vi "Measurement UI.vi"() -> ()   [LabVIEW 2021, in "Table and Multicolumn Listbox.lvlib"]
uses:
  Table and Multicolumn Listbox.lvlib
panel:
  in  "Tab Control":enum32{"Table", "Multicolumn Listbox"}(tab)
  out "Table":string[][](table)
  out "Multicolumn Listbox":i32(listbox)
  in  "Value to be Inserted":string
  in  "Update":bool
  in  "Cell Coordinates":cluster{"Row":i32, "Column":i32}
  in  "Clear":bool
  # "Source: https://forums.ni.com/t5/Example-Code/Programmatically-Write-Values-to-a-Multicolumn-Listbox/ta-p/3495593"
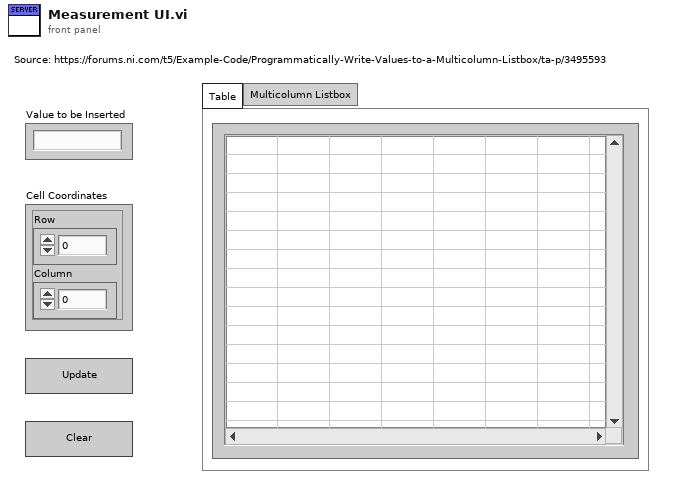
[diagram p1: front panel]
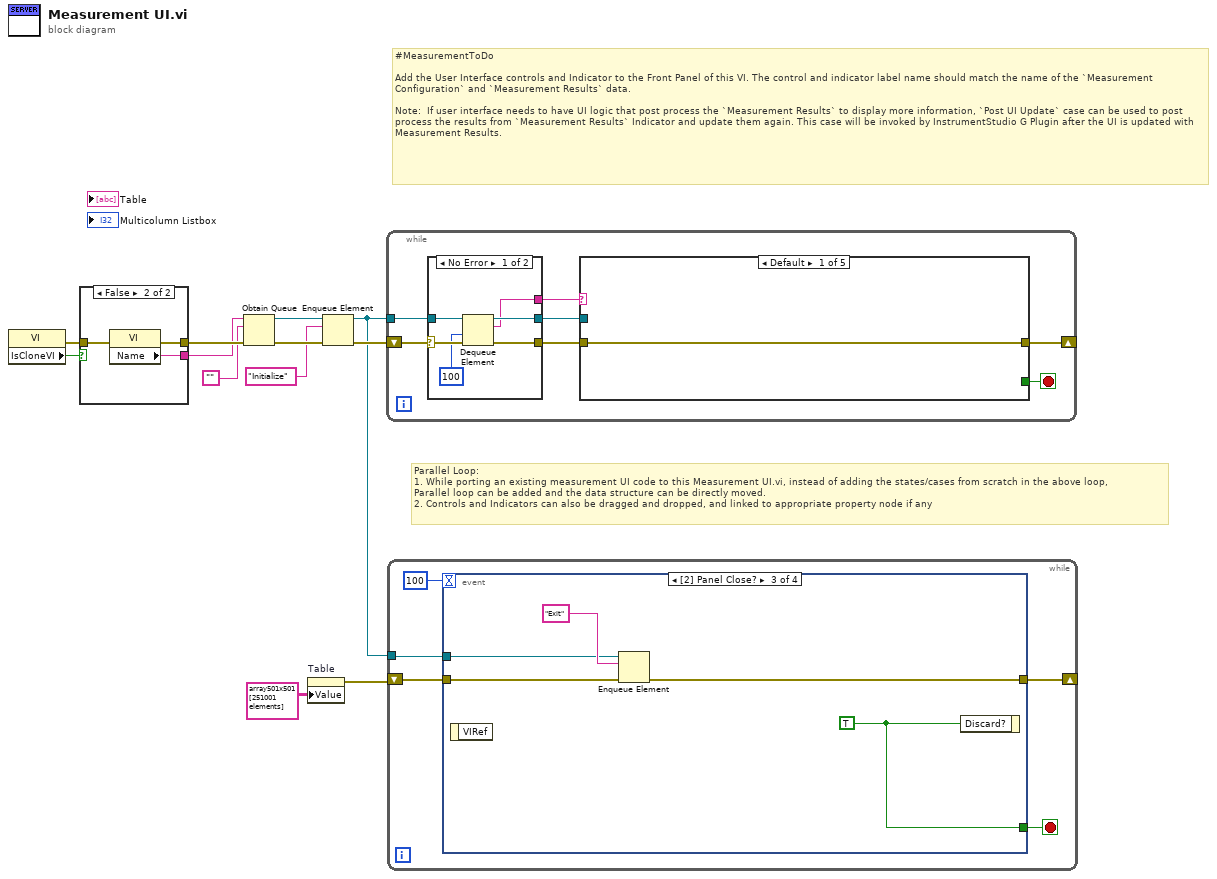
[diagram p0: block diagram]
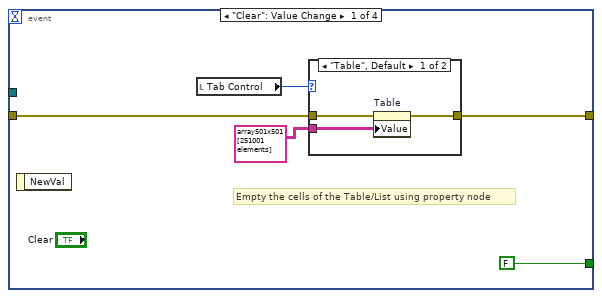
[diagram p2: hidden frame]
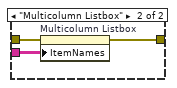
[diagram p3: hidden frame]
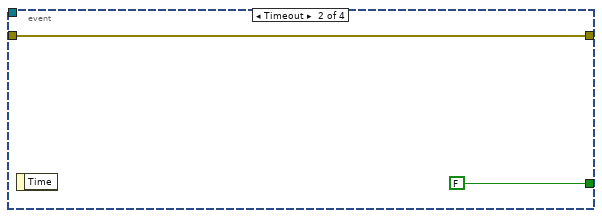
[diagram p4: hidden frame]
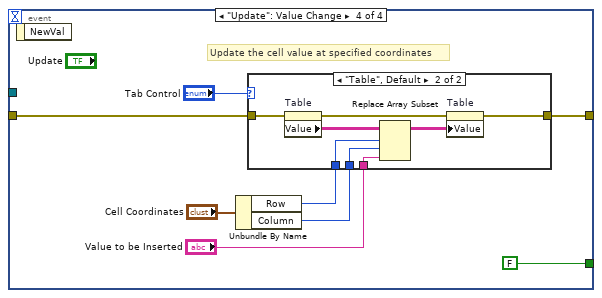
[diagram p5: hidden frame]
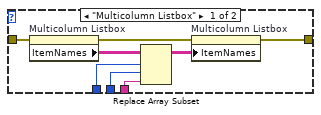
[diagram p6: hidden frame]
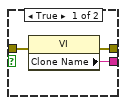
[diagram p7: hidden frame]
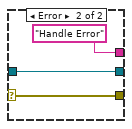
[diagram p8: hidden frame]
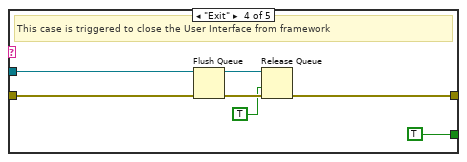
[diagram p11: hidden frame]
diagram:
  # "Parallel Loop:\n1. While porting an existing measurement UI code to this Measurement UI.vi, instead of adding the states/cases from scratch in the above loop,\nParallel loop can be added and the data structure can be directly moved.\n2. Controls and Indicators can also be dragged and dropped, and linked to appropriate property node if any"
  # "#MeasurementToDo  \n\nAdd the User Interface controls and Indicator to the Front Panel of this VI. The control and indicator label name should match the name of the `Measurement Configuration` and `Measurement Results` data.\n\nNote:  If user interface needs to have UI logic that post process the `Measurement Results` to display more information, `Post UI Update` case can be used to post process the results from `Measurement Results` Indicator and update them again. This case will be invoked by InstrumentStudio G Plugin after the UI is updated with Measurement Results."
  n1 = property class="VI"() -> (error out=w4:errorcluster, "IsCloneVI"=w5:bool)  [unwired: 2 in, 1 out]
  n2 = case shown="False" w5 {
    tunnel: [w15 w18] -> w12
    tunnel: [w14 w17] -> w11
    tunnel: w4 -> [w13 w16]
    frame True {
      n3 = property class="VI"(error in=w13) -> (error out=w15:errorcluster, "Clone Name"=w14:string)  [unwired: 1 in, 1 out]
    }
    frame False {
      n4 = property class="VI"(error in=w16) -> (error out=w18:errorcluster, "Name"=w17:string)  [unwired: 1 in, 1 out]
    }
  }
  n5 = Obtain Queue(name (unnamed)=w11, element data type="", error in (no error)=w12) -> (queue out=w8:refnum<queue>, error out=w10:errorcluster)  [unwired: 2 in, 1 out]
  n6 = property on="Table" class="Tbl (strict)"("Value"=string[][] array501x501[251001 elements] ("Table")) -> (error out=w2:errorcluster)  [unwired: 2 in, 1 out]
  n7 = Enqueue Element(queue=w8, element="Initialize", error in (no error)=w10) -> (queue out=w3:refnum<queue>, error out=w9:errorcluster)  [unwired: 1 in, 1 out]
  n8 = while {
    shift-right: [w20] -> _
    shift-left: w9 -> [w25]
    tunnel: w3 -> [w23]
    stop <- w19 stop-if-true
    n9 = case shown="No Error" w25 {
      selector: w25 -> [w31 w34]
      tunnel: [w30 w34] -> w24
      tunnel: w23 -> [w29 w33]
      tunnel: [w28 w33] -> w22
      tunnel: [w27 "Handle Error"] -> w21
      frame No Error {
        n10 = Dequeue Element(queue=w29, timeout in ms (-1)=100, error in (no error)=w31) -> (queue out=w28:refnum<queue>, element=w27:string, error out=w30:errorcluster)  [unwired: 1 out]
      }
      frame Error {
      }
    }
    n11 = case shown="Default" w21 {
      tunnel: w24 -> [w35 w36 w37 w44 w45]
      tunnel: w22 -> [_ _ _ w42 _]
      tunnel: [w35 w36 w37 w39 w45] -> w20
      tunnel: [_ _ _ TRUE _] -> w19
      frame Default {
      }
      frame "Initialize" {
      }
      frame "Post UI Update" {
        # "This case will be triggered, after framework updates the User interface with result values."
      }
      frame "Exit" {
        # "This case is triggered to close the User Interface from framework"
        n12 = Flush Queue(queue=w42, error in (no error)=w44) -> (queue out=w41:refnum<queue>, error out=w40:errorcluster)  [unwired: 1 out]
        n13 = Release Queue(queue=w41, force destroy? (F)=TRUE, error in (no error)=w40) -> (error out=w39:errorcluster)  [unwired: 2 out]
      }
      frame "Handle Error" {
      }
    }
  }
  n14 = while {
    tunnel: w3 -> [w46]
    shift-right: [w48] -> _
    shift-left: w2 -> [w49]
    stop <- w50 stop-if-true
    n15 = event shown="[2] Panel Close?" {
      selector: _ -> [_ _ _ _]
      dyn-events: _ -> [_ _ _ _]
      timeout: 100 -> [_ _ _ _]
      tunnel: [FALSE FALSE ("Discard?") w68 FALSE] -> w50
      tunnel: w49 -> [w53 w63 w65 w71]
      tunnel: [w52 w63 w64 w70] -> w48
      tunnel: w46 -> [_ _ w66 _]
      event "Clear": Value Change {
        # "Empty the cells of the Table/List using property node"
        n16 = event-data() -> ()  [unwired: 1 in, 1 out]
        n17 = local read "Tab Control"() -> (w51:enum32{"Table", "Multicolumn Listbox"})
        n18 = case shown="\"Table\", Default" w51 {
          tunnel: string[][] array501x501[251001 elements] ("Item Names") -> [w58 w61]
          tunnel: w53 -> [w57 w60]
          tunnel: [w56 w59] -> w52
          frame "Table", Default {
            n19 = property on="Table" class="Tbl (strict)"(error in=w57, "Value"=w58) -> (error out=w56:errorcluster)  [unwired: 1 in, 1 out]
          }
          frame "Multicolumn Listbox" {
            n20 = property on="Multicolumn Listbox" class="MCListbox (strict)"(error in=w60, "ItemNames"=w61) -> (error out=w59:errorcluster)  [unwired: 1 in, 1 out]
          }
        }
      }
      event Timeout {
        n21 = event-data() -> ()  [unwired: 1 in, 1 out]
      }
      event Panel Close? {
        w68 = TRUE ("Discard?")
        n22 = event-data() -> ()  [unwired: 1 in, 1 out]
        n23 = Enqueue Element(queue=w66, element="Exit", error in (no error)=w65) -> (error out=w64:errorcluster)  [unwired: 1 in, 2 out]
        n24 = event-data("Discard?"=w68) -> ()  [unwired: 1 in, 1 out]
      }
      event "Update": Value Change {
        # "Update the cell value at specified coordinates"
        n25 = event-data() -> ()  [unwired: 1 in, 1 out]
        n26 = Unbundle By Name("Cell Coordinates") -> ("Row"=w74:i32, "Column"=w75:i32)
        n27 = case shown="\"Table\", Default" "Tab Control" {
          tunnel: "Value to be Inserted" -> [w83 w91]
          tunnel: w75 -> [w82 w90]
          tunnel: w74 -> [w80 w88]
          tunnel: w71 -> [w79 w87]
          tunnel: [w77 w85] -> w70
          frame "Multicolumn Listbox" {
            n28 = property on="Multicolumn Listbox" class="MCListbox (strict)"(error in=w79) -> (error out=w78:errorcluster, "ItemNames"=w81:string[][])  [unwired: 1 in, 1 out]
            n29 = Replace Array Subset(array=w81, new element=w83, index (row)=w80, index (col)=w82) -> (w84:string[][])
            n30 = property on="Multicolumn Listbox" class="MCListbox (strict)"(error in=w78, "ItemNames"=w84) -> (error out=w77:errorcluster)  [unwired: 1 in, 1 out]
          }
          frame "Table", Default {
            n31 = property on="Table" class="Tbl (strict)"(error in=w87) -> (error out=w86:errorcluster, "Value"=w89:string[][])  [unwired: 1 in, 1 out]
            n32 = Replace Array Subset(array=w89, new element=w91, index (row)=w88, index (col)=w90) -> (w92:string[][])
            n33 = property on="Table" class="Tbl (strict)"(error in=w86, "Value"=w92) -> (error out=w85:errorcluster)  [unwired: 1 in, 1 out]
          }
        }
      }
    }
  }
